vi "test waveform graph updates.vi"() -> ()   [LabVIEW 2017]
doc: "Developed by Kevin Thompson\nkevin@thompsonengineering.net\n\nCopyright 2018-2020\nThompson Engineering, LLC"
panel:
  out "XY Graph":cluster{dbl[], dbl[]}[](graph)=[{[0.0, 1.0, 2.0, 3.0, 4.0, 5.0, 6.0, 7.0, 8.0, 9.0, 10.0, 11.0, 12.0, 13.0, 14.0, 15.0, 16.0, 17.0, 18.0, 19.0, 20.0, 21.0, 22.0, 23.0, 24.0, 25.0, 26.0, 27.0, 28.0, 29.0, 30.0, 31.0, 32.0, 33.0, 34.0, 35.0, 36.0, 37.0, 38.0, 39.0, 40.0, 41.0, 42.0, 43.0, 44.0, 45.0, 46.0, 47.0, 48.0, 49.0, 50.0, 51.0, 52.0, 53.0, 54.0, 55.0, 56.0, 57.0, 58.0, 59.0, 60.0, 61.0, 62.0, 63.0, 64.0, 65.0, 66.0, 67.0, 68.0, 69.0, 70.0, 71.0, 72.0, 73.0, 74.0, 75.0, 76.0, 77.0, 78.0, 79.0, 80.0, 81.0, 82.0, 83.0, 84.0, 85.0, 86.0, 87.0, 88.0, 89.0, 90.0, 91.0, 92.0, 93.0, 94.0, 95.0, 96.0, 97.0, 98.0, 99.0, 100.0, 101.0, 102.0, 103.0, 104.0, 105.0, 106.0, 107.0, 108.0, 109.0, 110.0, 111.0, 112.0, 113.0, 114.0, 115.0, 116.0, 117.0, 118.0, 119.0, 120.0, 121.0, 122.0, 123.0, 124.0, 125.0, 126.0, 127.0, 128.0, 129.0, 130.0, 131.0, 132.0, 133.0, 134.0, 135.0, 136.0, 137.0, 138.0, 139.0, 140.0, 141.0, 142.0, 143.0, 144.0, 145.0, 146.0, 147.0, 148.0, 149.0, 150.0, 151.0, 152.0, 153.0, 154.0, 155.0, 156.0, 157.0, 158.0, 159.0, 160.0, 161.0, 162.0, 163.0, 164.0, 165.0, 166.0, 167.0, 168.0, 169.0, 170.0, 171.0, 172.0, 173.0, 174.0, 175.0, 176.0, 177.0, 178.0, 179.0, 180.0, 181.0, 182.0, 183.0, 184.0, 185.0, 186.0, 187.0, 188.0, 189.0, 190.0, 191.0, 192.0, 193.0, 194.0, 195.0, 196.0, 197.0, 198.0, 199.0, 200.0, 201.0, 202.0, 203.0, 204.0, 205.0, 206.0, 207.0, 208.0, 209.0, 210.0, 211.0, 212.0, 213.0, 214.0, 215.0, 216.0, 217.0, 218.0, 219.0, 220.0, 221.0, 222.0, 223.0, 224.0, 225.0, 226.0, 227.0, 228.0, 229.0, 230.0, 231.0, 232.0, 233.0, 234.0, 235.0, 236.0, 237.0, 238.0, 239.0, 240.0, 241.0, 242.0, 243.0, 244.0, 245.0, 246.0, 247.0, 248.0, 249.0, 250.0, 251.0, 252.0, 253.0, 254.0, 255.0, 256.0, 257.0, 258.0, 259.0, 260.0, 261.0, 262.0, 263.0, 264.0, 265.0, 266.0, 267.0, 268.0, 269.0, 270.0, 271.0, 272.0, 273.0, 274.0, 275.0, 276.0, 277.0, 278.0, 279.0, 280.0, 281.0, 282.0, 283.0, 284.0, 285.0, 286.0, 287.0, 288.0, 289.0, 290.0, 291.0, 292.0, 293.0, 294.0, 295.0, 296.0, 297.0, 298.0, 299.0, 300.0, 301.0, 302.0, 303.0, 304.0, 305.0, 306.0, 307.0, 308.0, 309.0, 310.0, 311.0, 312.0, 313.0, 314.0, 315.0, 316.0, 317.0, 318.0, 319.0, 320.0, 321.0, 322.0, 323.0, 324.0, 325.0, 326.0, 327.0, 328.0, 329.0, 330.0, 331.0, 332.0, 333.0, 334.0, 335.0, 336.0, 337.0, 338.0, 339.0, 340.0, 341.0, 342.0, 343.0, 344.0, 345.0, 346.0, 347.0, 348.0, 349.0, 350.0, 351.0, 352.0, 353.0, 354.0, 355.0, 356.0, 357.0, 358.0, 359.0], [0.0, 0.24740395925452294, 0.479425538604203, 0.6816387600233341, 0.8414709848078965, 0.9489846193555862, 0.9974949866040544, 0.9839859468739369, 0.9092974268256817, 0.7780731968879212, 0.5984721441039564, 0.38166099205233167, 0.1411200080598672, -0.10819513453010837, -0.35078322768961984, -0.5715613187423437, -0.7568024953079282, -0.8949893582285835, -0.977530117665097, -0.999292788975378, -0.9589242746631385, -0.858934493426592, -0.7055403255703919, -0.5082790774992584, -0.27941549819892586, -0.03317921654755682, 0.21511998808781552, 0.4500440737806176, 0.6569865987187891, 0.8230808790115055, 0.9379999767747389, 0.9945987791111761, 0.9893582466233818, 0.9226042102393402, 0.7984871126234903, 0.6247239537541924, 0.4121184852417566, 0.17388948538043356, -0.0751511204618093, -0.31951919362227366, -0.5440211108893698, -0.7346984304047954, -0.87969575997167, -0.9699978679206785, -0.9999902065507035, -0.9678079975112615, -0.8754521746884285, -0.72866497582717, -0.5365729180004349, -0.3111193549811273, -0.06632189735120068, 0.182599134631134, 0.4201670368266409, 0.6316109877182386, 0.803784426551621, 0.9259824428086272, 0.9906073556948704, 0.9936411011327626, 0.934895055524683, 0.8180217634546941, 0.6502878401571168, 0.4421221685765394, 0.2064674819377966, -0.04202435271884079, -0.2879033166650653, -0.5158818468181093, -0.711785342369123, -0.8634334728079056, -0.9613974918795568, -0.9995864713592172, -0.9756260054681576, -0.8910058399248534, -0.750987246771676, -0.5642759039618552, -0.34248061846961253, -0.09939154689884817, 0.14987720966295234, 0.3898273272463786, 0.605539869719601, 0.7836028759783553, 0.9129452507276277, 0.9855251115651197, 0.9968297942787993, 0.9461564284508708, 0.8366556385360561, 0.675135653292801, 0.47163900309419615, 0.23881812402958275, -0.008851309290403876, -0.25597041106933305, -0.4871745124605095, -0.6880884622582969, -0.8462204041751706, -0.9517384599623535, -0.9980820279793963, -0.9823696896284233, -0.9055783620066239, -0.7724825579327704, -0.5913575298651244, -0.3734647547841147, -0.13235175009777303, 0.11699024537436405, 0.3590583540221683, 0.5788019532877502, 0.7625584504796027, 0.8989027566124672, 0.979357643103917, 0.9989208147888241, 0.956375928404503, 0.8543682189235223, 0.6992400316550977, 0.500636485932415, 0.27090578830786904, 0.02433148087720227, -0.22375564018679642, -0.45793071928681145, -0.6636338842129675, -0.8280755084772445, -0.9410314083429535, -0.9954785330494551, -0.9880316240928618, -0.9191536942035773, -0.7931272394572851, -0.617787974410896, -0.404037645323065, -0.165166212373579, 0.08397445569174683, 0.3278939988258263, 0.5514266812416906, 0.740674323409674, 0.8838704235458307, 0.9721117417027341, 0.9999118601072672, 0.9655423020447212, 0.8711400001691764, 0.7225744323811351, 0.5290826861200238, 0.30269514100631545, 0.057487478104924564, -0.1912944777489552, -0.428182669496151, -0.6384485367231334, -0.8090187662119065, -0.929288127236339, -0.9917788534431158, -0.9926055741456128, -0.9317168878547055, -0.8128985581744033, -0.6435381333569995, -0.4341656243337532, -0.19779879963646227, 0.050866196399306694, 0.2963685787093853, 0.523444198233198, 0.7179745927716441, 0.8678648045849774, 0.9637953862840878, 0.9998018389311463, 0.9736454556949781, 0.8869525137988248, 0.7451131604793488, 0.5569462797382114, 0.33415117684842055, 0.09058017221711874, -0.158622668804709, -0.397963120556671, -0.6125601529754697, -0.78907116196914, -0.9165215479156338, -0.9869870631127111, -0.996086503119594, -0.943254108829076, -0.8317747426285983, -0.6685796515669709, -0.46381551598382736, -0.23021357807075407, 0.017701925105413577, 0.2645168083164075, 0.4948853175526281, 0.6944842546815092, 0.8509035245341184, 0.9544177345154423, 0.9985908724117705, 0.9806764664578257, 0.9017883476488092, 0.7668313971238714, 0.5841965844132856, 0.365239257594056, 0.123573122745224, -0.1257761903592125, -0.36730534913419133, -0.5859972403145538, -0.7682546613236668, -0.9027457284726567, -0.981108438603097, -0.9984705779426957, -0.9537526527594719, -0.8497350070535673, -0.6928849542336957, -0.4929546708933114, -0.26237485370392877, -0.015481838903188173, 0.23237376165548454, 0.46578148719844353, 0.6702291758433747, 0.833005260536624, 0.9439891127251193, 0.9962802940213323, 0.9866275920404853, 0.9156311650396451, 0.7877052269841179, 0.6108035931029845, 0.39592515018183416, 0.15642999905467883, -0.09279121175730869, -0.3362431144491573, -0.5587890488516163, -0.7465921866472573, -0.8879758383376634, -0.9741494532413135, -0.9997551733586199, -0.9632009590319782, -0.8667595742607592, -0.7164272772437812, -0.5215510020869119, -0.2942472117115055, -0.04864855487508726, 0.19997483347801748, 0.43616475524782494, 0.645236065065984, 0.8141897215084345, 0.9325210045313215, 0.9928726480845371, 0.9914922792803779, 0.9284657227653786, 0.8077116645594764, 0.6367380071391379, 0.42617506442530745, 0.18911462035089152, -0.05970405485516448, -0.3048106211022167, -0.5309655392553846, -0.7241075918674496, -0.8722281415753229, -0.9661177700083929, -0.9999388748177166, -0.9715886235161092, -0.8828296974172939, -0.7391806966492228, -0.5495730203270262, -0.32579555541456173, -0.08176170083154902, 0.16735570030280691, 0.4060677345664961, 0.6195324438519512, 0.79447762643532, 0.9200260381967906, 0.9883716869768853, 0.9952651713612277, 0.9402778878788489, 0.8268286794901034, 0.6619712684902924, 0.45595569022148996, 0.22159099552021236, -0.026551154023966794, -0.2730424814093603, -0.5025573497604873, -0.7008256362004742, -0.8555199789753223, -0.9570222331011646, -0.999021480034635, -0.9789064100214568, -0.8979276806892913, -0.7611201572139108, -0.5769898687885426, -0.3569851449269173, -0.11478481378318722, 0.13455228113037063, 0.375523566896625, 0.5931466160920859, 0.7738906815578891, 0.9065179727230256, 0.9827823669926928, 0.9979421137117938, 0.9510546532543747, 0.8450352208159536, 0.6864755912087755, 0.48523423423072903, 0.25382336276203626, 0.006630983970279104, -0.2409736772881011, -0.47359576242974594, -0.6767719568873076, -0.8378697489573207, -0.9468728581933475, -0.9970039992110719, -0.9851462604682474, -0.9120368987278785, -0.7822215000035424, -0.6037713570372523, -0.38778163540943045, -0.1476815298816789, 0.1016006978902495, 0.3445658863623454, 0.5661076368981803, 0.7524515564694672, 0.8920116826993705, 0.9761108428874015, 0.9995201585807313, 0.9607841519107266, 0.862311240157329, 0.7102239920275675, 0.5139784559875352, 0.2857762289683941, 0.039805820166669656, -0.20863952173666145, -0.4441126687075084, -0.651973040962877, -0.8192968873112808, -0.9356808214066555, -0.9938886539233752, -0.9903013037606052, -0.9251418149764185, -0.8024614889885606, -0.6298879942744539, -0.4181511148892831, -0.1804156244623088, 0.06853723566485535, 0.31322878243308516, 0.5384452806085791, 0.7301838591531669, 0.8765231419236595, 0.9683644611001854, 0.9999975682825487, 0.9694556700786149, 0.8786377137914245, 0.7331903200732922, 0.542156703402608, 0.31741440880766936, 0.07293682364477497, -0.1760756199485871, -0.4141405343019522, -0.6264561960895026, -0.799821845795485, -0.9234584470040598, -0.9896788746762244, -0.9943658633527529, -0.9372279987787994, -0.8218178366308225, -0.6553110218111473, -0.44806014160260915, -0.2129510519332497, 0.03539830273366068, 0.2815467623854851, 0.5101900080017631, 0.7071121099856378, 0.8600694058124533, 0.9595517516643209, 0.9993738171110836, 0.9770596589983012]}, ...(2 in all)]
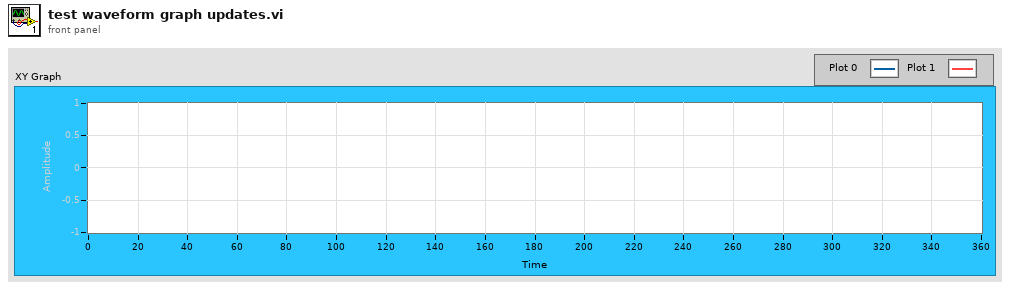
[diagram p1: front panel]
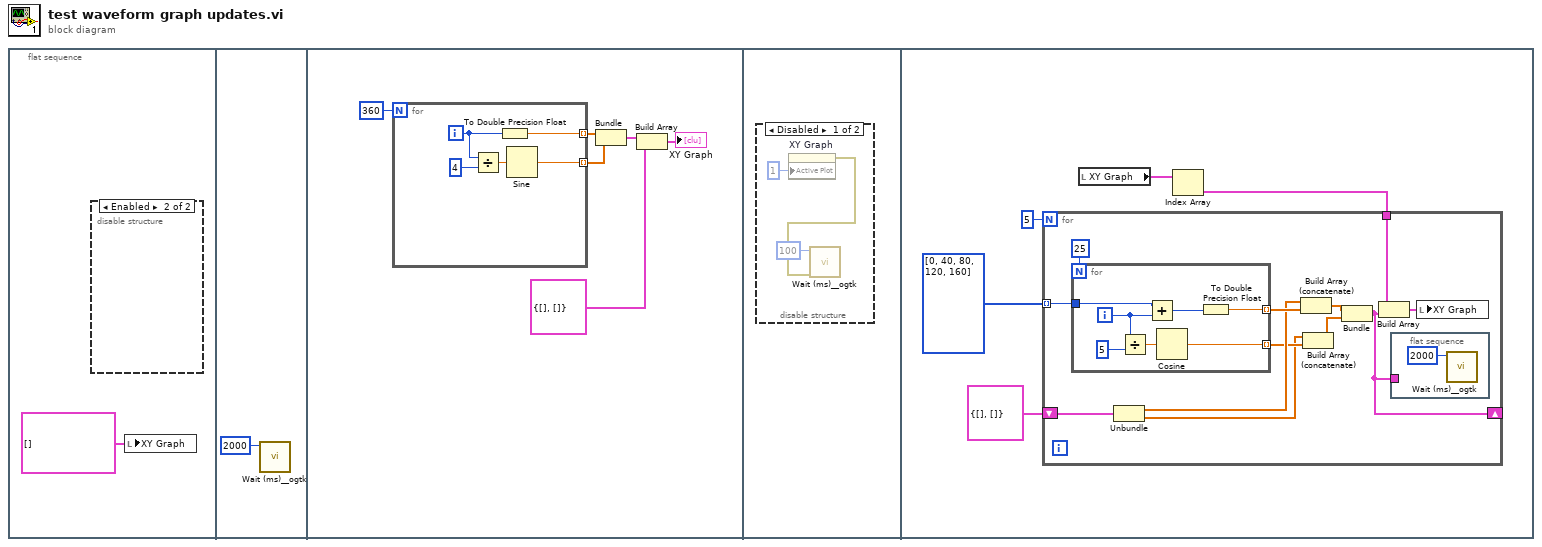
[diagram p0: block diagram]
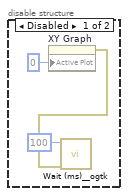
[diagram p2: hidden frame]
diagram:
  n1 = flat-sequence {
    frame #0 {
      n2 = disable-structure shown="Enabled" {
        frame Disabled {
          n3 = property on="XY Graph" class="XYGraph (strict)"("Active Plot"=u32 0) -> (error out=w2:errorcluster)  [unwired: 2 in, 1 out]
          n4 = call <userlib>:"Wait (ms)__ogtk.vi"("error in (no error)"=w2, "milliseconds to wait"=u32 100) -> ()  [unwired: 8 in, 2 out]
        }
        frame Enabled {
        }
      }
      n5 = local write "XY Graph"(cluster{dbl[], dbl[]}[] [] ("XY Graph")) -> ()
    }
    frame #1 {
      n6 = call <userlib>:"Wait (ms)__ogtk.vi"("milliseconds to wait"=u32 2000) -> ()  [unwired: 9 in, 2 out]
    }
    frame #2 {
      n7 = for {
        N: 360 -> [_]
        tunnel: [w14] -> w9 mode=indexing
        tunnel: [w12] -> w10 mode=indexing
        i -> [w13]
        n8 = Divide(x=w13, y=4) -> (x/y=w16:dbl)
        n9 = To Double Precision Float(number=w13) -> (double precision float=w12:dbl)
        n10 = Sine(x=w16) -> (sin(x)=w14:dbl)
      }
      n11 = Bundle(w10, w9) -> (w8:cluster{dbl[], dbl[]})  [unwired: 1 in]
      n12 = Build Array(w8, cluster{dbl[], dbl[]} {[], []} ("output cluster")) -> (→"XY Graph":cluster{dbl[], dbl[]}[])
    }
    frame #3 {
      n13 = disable-structure shown="Disabled" {
        frame Disabled {
          n14 = property on="XY Graph" class="XYGraph (strict)"("Active Plot"=u32 1) -> (error out=w18:errorcluster)  [unwired: 2 in, 1 out]
          n15 = call <userlib>:"Wait (ms)__ogtk.vi"("error in (no error)"=w18, "milliseconds to wait"=u32 100) -> ()  [unwired: 8 in, 2 out]
        }
        frame Enabled {
        }
      }
    }
    frame #4 {
      n16 = local read "XY Graph"() -> (w22:cluster{dbl[], dbl[]}[])
      n17 = Index Array(array=w22) -> (element=w21:cluster{dbl[], dbl[]})  [unwired: 1 in]
      n18 = for {
        N: 5 -> [_]
        tunnel: i32[] [0, 40, 80, 120, 160] -> [w35] mode=indexing
        tunnel: w21 -> [w33]
        shift-right: [w25] -> _
        shift-left: cluster{dbl[], dbl[]} {[], []} ("output cluster") -> [w32]
        n19 = for {
          N: 25 -> [_]
          tunnel: [w42] -> w31 mode=indexing
          tunnel: [w41] -> w29 mode=indexing
          tunnel: w35 -> [w39]
          i -> [w40]
          n20 = Divide(x=w40, y=5) -> (x/y=w44:dbl)
          n21 = Add(x=w39, y=w40) -> (x+y=w38:i32)
          n22 = Cosine(x=w44) -> (cos(x)=w41:dbl)
          n23 = To Double Precision Float(number=w38) -> (double precision float=w42:dbl)
        }
        n24 = Unbundle(w32) -> (w30:dbl[], w28:dbl[])
        n25 = Build Array (concatenate)(w30, w31) -> (w27:dbl[])
        n26 = Build Array (concatenate)(w28, w29) -> (w26:dbl[])
        n27 = Bundle(w27, w26) -> (w25:cluster{dbl[], dbl[]})  [unwired: 1 in]
        n28 = Build Array(w33, w25) -> (w34:cluster{dbl[], dbl[]}[])
        n29 = flat-sequence {
          tunnel: w25 -> [_]
          frame #0 {
            n30 = call <userlib>:"Wait (ms)__ogtk.vi"("milliseconds to wait"=u32 2000) -> ()  [unwired: 9 in, 2 out]
          }
        }
        n31 = local write "XY Graph"(w34) -> ()
      }
    }
  }
